vi "Calc_Brightness_Metric_SLM.vi"(11 "Image In":dbl[][](array[numeric])) -> (3 "Brightness":dbl)   [LabVIEW 2014]
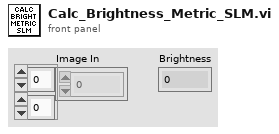
[diagram p1: front panel]
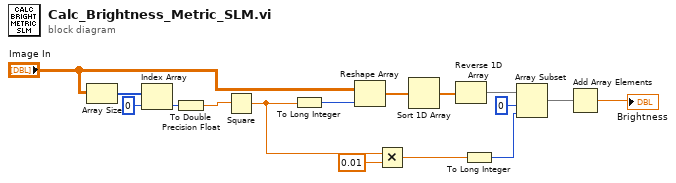
[diagram p0: block diagram]
diagram:
  n1 = Array Size(array="Image In") -> (size(s)=w1:i32[])
  n2 = Index Array(array=w1, index=0) -> (element=w3:i32)
  n3 = To Double Precision Float(number=w3) -> (double precision float=w6:dbl)
  n4 = Square(x=w6) -> (x^2=w9:dbl)
  n5 = To Long Integer(number=w9) -> (32bit integer=w5:i32)
  n6 = Reshape Array("Image In", w5) -> (w7:dbl[])
  n7 = Multiply(x=w9, y=0.01) -> (x*y=w13:dbl)
  n8 = Sort 1D Array(array=w7) -> (sorted array=w8:dbl[])
  n9 = Reverse 1D Array(array=w8) -> (reversed array=w11:dbl[])
  n10 = To Long Integer(number=w13) -> (32bit integer=w14:i32)
  n11 = Array Subset(array=w11, index=0, length=w14) -> (w15:dbl[])
  n12 = Add Array Elements(numeric array=w15) -> (sum=→"Brightness":dbl)
